vi "CaptureImageLinux.vi"(8 "error in":errorcluster, 10 "WindowName":string="Untitled 3 Front Panel *", 11 "PathWheretoSave":string="/home/lvadmin/inmathed_linux_GUI/inmathed_linux_GUI/LabVIEWTestSystems/LV GUI ToolKit/LV GUI 2013/LabVIEW GUI Automation Toolkit/Utility/Linux VIs/1.jpg") -> (0 "error out":errorcluster)   [LabVIEW 2013]
uses:
  <vilib>/Utility/file.llb/Read From Spreadsheet File (I64).vi
  <vilib>/picture/picture.llb/Draw True-Color Pixmap.vi
panel:
  out "new picture":picture
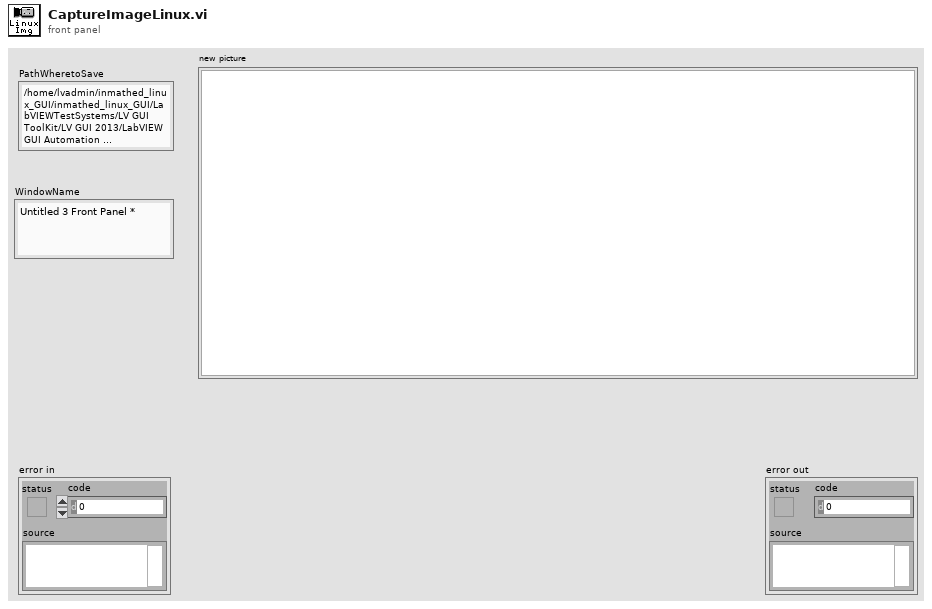
[diagram p1: front panel]
types:
  T1 = typedef "imagedata.ctl" = cluster{"image type":i32, "image depth":i32, "image":u8[], "mask":u8[], "colors":u32[], "Rectangle":cluster{"left":i16, "top":i16, "right":i16, "bottom":i16}}
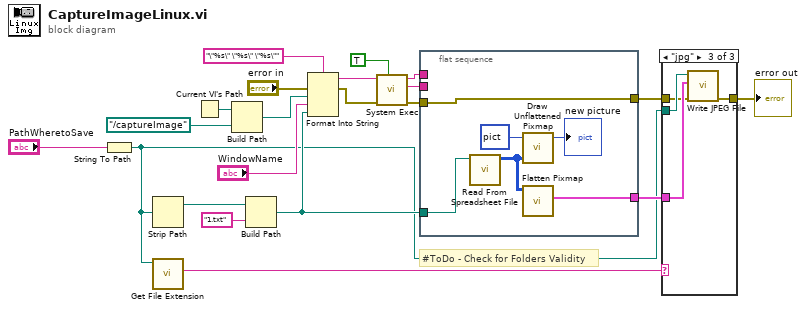
[diagram p0: block diagram]
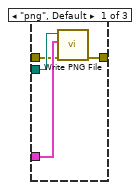
[diagram p2: hidden frame]
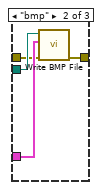
[diagram p3: hidden frame]
diagram:
  # "#ToDo - Check for Folders Validity"
  n1 = String To Path(string="PathWheretoSave") -> (path=w6:path)
  n2 = Strip Path(path=w6) -> (stripped path=w14:path)  [unwired: 1 out]
  n3 = call <vilib>:"Get File Extension.vi"("file"=w6) -> ("lowercase file extension"=w15:string)  [unwired: 7 in, 3 out]
  n4 = Current VI's Path() -> (path=w3:path)
  n5 = Build Path(base path=w3, name or relative path=path "../captureImage" ("path")) -> (appended path=w1:path)
  n6 = Build Path(base path=w14, name or relative path="1.txt") -> (appended path=w12:path)
  n7 = Format Into String(format string="\"%s\" \"%s\" \"%s\"", error in="error in", w1, "WindowName", w12) -> (resulting string=w18:string, error out=w17:errorcluster)  [unwired: 1 in]
  n8 = call <vilib>:"System Exec.vi"("wait until completion? (T)"=TRUE, "error in (no error)"=w17, "command line"=w18) -> ("error out"=w11:errorcluster, "standard error"=w7:string, "standard output"=w8:string)  [unwired: 5 in, 1 out]
  n9 = flat-sequence {
    tunnel: [w25] -> w16
    tunnel: w12 -> [w24]
    tunnel: [w23] -> w10
    tunnel: w11 -> [w23]
    tunnel: w8 -> [_]
    tunnel: w7 -> [_]
    frame #0 {
      n10 = call-poly <vilib>:"Read From Spreadsheet File.vi"("file path (dialog if empty)"=w24) -> ("all rows"=w26:i64[][])  [unwired: 6 in, 4 out]
      n11 = call-poly <vilib>:"Draw Unflattened Pixmap.vi"("picture"=picture data[5B], "data (RGB format)"=w26) -> ("new picture"=→"new picture":picture)  [unwired: 7 in]
      n12 = call <vilib>:"Flatten Pixmap.vi"("24-bit pixmap"=w26) -> ("image data"=w25:T1)  [unwired: 10 in]
    }
  }
  n13 = case shown="\"jpg\"" w15 {
    tunnel: w16 -> [w30 w34 w39]
    tunnel: w6 -> [w31 w35 w38]
    tunnel: w10 -> [w29 w33 w37]
    tunnel: [w28 w32 w36] -> w5
    frame "png", Default {
      n14 = call <vilib>:"Write PNG File.vi"("error in (no error)"=w29, "image data"=w30, "path to PNG file"=w31) -> ("error out"=w28:errorcluster)  [unwired: 7 in, 1 out]
    }
    frame "bmp" {
      n15 = call <vilib>:"Write BMP File.vi"("error in (no error)"=w33, "image data"=w34, "path to BMP file"=w35) -> ("error out"=w32:errorcluster)  [unwired: 7 in, 1 out]
    }
    frame "jpg" {
      n16 = call <vilib>:"Write JPEG File.vi"("error in (no error)"=w37, "image data"=w39, "path to JPEG file"=w38) -> ("error out"=w36:errorcluster)  [unwired: 7 in, 1 out]
    }
  }
  "error out" <- w5
